vi "maintenance.vi"(8 "errorIn":errorcluster, 9 "status":bool, 11 "errorLocation":string) -> (0 "errorOut":errorcluster)   [LabVIEW 2020, in "maintenanceLibrary.lvlib"]
uses:
  maintenanceLibrary.lvlib
  databaseLibrary.lvlib
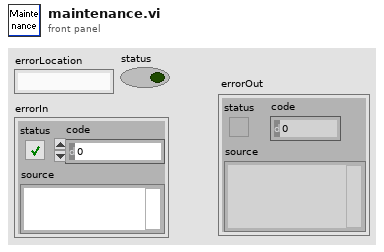
[diagram p1: front panel]
types:
  T1 = cluster{"date":string, "time":string, "errorID":i32, "errorLocation":string, "description":string}
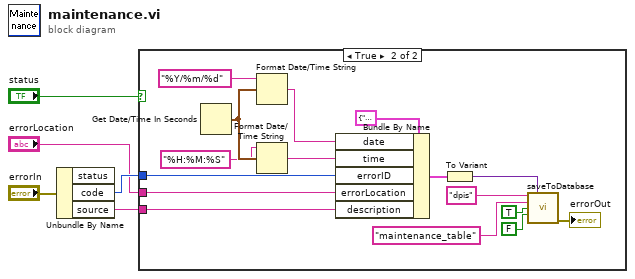
[diagram p0: block diagram]
diagram:
  n1 = Unbundle By Name("errorIn") -> ("code"=w5:i32, "source"=w3:string)  [unwired: 1 out]
  n2 = case shown="True" "status" {
    tunnel: w5 -> [_ w15]
    tunnel: "errorLocation" -> [_ w14]
    tunnel: w3 -> [_ w13]
    frame False {
    }
    frame True {
      n3 = Get Date/Time In Seconds() -> (seconds since 1Jan1904=w20:timestamp)
      n4 = Format Date/Time String(time format string (%c)="%Y/%m/%d", seconds (now)=w20) -> (date/time string=w17:string)  [unwired: 1 in]
      n5 = Format Date/Time String(time format string (%c)="%H:%M:%S", seconds (now)=w20) -> (date/time string=w16:string)  [unwired: 1 in]
      n6 = Bundle By Name(cluster=T1 {"date"="", "time"="", "errorID"=0, "errorLocation"="", "description"=""}, "date"=w17, "time"=w16, "errorID"=w15, "errorLocation"=w14, "description"=w13) -> (w12:T1)
      n7 = To Variant(anything=w12) -> (Variant=w11:variant)
      n8 = call "saveToDatabase.vi"("Connection"="dpis", "Data"=w11, "Table"="maintenance_table", "Auto Increment ID?"=TRUE, "Delete row?"=FALSE) -> ("Error out"=→"errorOut":errorcluster)  [unwired: 10 in]
    }
  }
